vi "WLAN - TV - OPPO - RW - UTIL - TestVectors_11N.vi"(0 "TV_IQComposite_11N":T1={"Standard"=3, "OFDM Advanced Controls"={"OFDM Auto Compute Acquisition Length Enabled"=0, "OFDM Maximum Symbols Used"=0, "OFDM Time Tracking Enabled"=0, "OFDM Channel Tracking Enabled"=0, "OFDM Amplitude Tracking Enabled"=1, "OFDM CFO Estimation Method"=0, "OFDM Phase Tracking Method"=0, "OFDM Header Detection Enabled"=0, "OFDM MAC FCS Check Enabled"=0, "#Avg"=10, "#Iterations"=10}, "Measurement Enabled"=FALSE, "#Packets"=0, "Guard Interval (s)"=0.0, "FEC Coding Type"=0, "80211n PLCP Frame Format"=0, "Generation Parameters"={"Channel Bandwidth(Hz)"=20000000.0, "MCS Index"=0, "OFDM Payload Length (bytes)"=4024, "Idle Interval(S)"=0.0}, "Power Level(dBm)"=0.0, "Center Frequency(Hz)"=0.0} {"Center Frequency(Hz)" format="%#_6p"; "Generation Parameters"."Channel Bandwidth(Hz)" items=["5M"=5000000.0, "10M"=10000000.0, "20M"=20000000.0, "40M"=40000000.0, "80M"=80000000.0, "160M"=160000000.0]; "80211n PLCP Frame Format" items=["Mixed Format", "Greenfield Format"]; "FEC Coding Type" items=["BCC", "LDPC"]; "OFDM Advanced Controls"."OFDM Phase Tracking Method" items=["Standard", "Instantaneous", "None", "Standard with Cubic Spline Fit"]; "OFDM Advanced Controls"."OFDM CFO Estimation Method" items=["Preamble Only", "Preamble and Data"]; "OFDM Advanced Controls"."OFDM Channel Tracking Enabled" items=["False", "True"]; "OFDM Advanced Controls"."OFDM Amplitude Tracking Enabled" items=["False", "True"]; "OFDM Advanced Controls"."OFDM Time Tracking Enabled" items=["True"=1, "False"=0]; "OFDM Advanced Controls"."OFDM Auto Compute Acquisition Length Enabled" items=["False", "True"]; "OFDM Advanced Controls"."OFDM MAC FCS Check Enabled" items=["False", "True"]; "OFDM Advanced Controls"."OFDM Header Detection Enabled" items=["False", "True"]; "Standard" items=["80211A/G/J/P OFDM", "80211B/G DSSS", "80211G DSSSOFDM", "80211N MIMOOFDM", "80211AC MIMOOFDM"]}, 7 "TV Paramaters":T3) -> (6 "TV":string[][](array[string]), 8 "Measure Config":string[][](array[string]))   [LabVIEW 2012]
uses:
  Includes/WLAN - TV - RW - INC - TV_Parameters.ctl
  Includes/WLAN - TV - OPPO - RW - INC - TV_IQComposite_11N.ctl
  Includes/WLAN - TV - RW - INC - TV_OFDM Demod.ctl
  Includes/WLAN - TV - RW - INC - Tx_Meas_Settings_OFDM_String.ctl
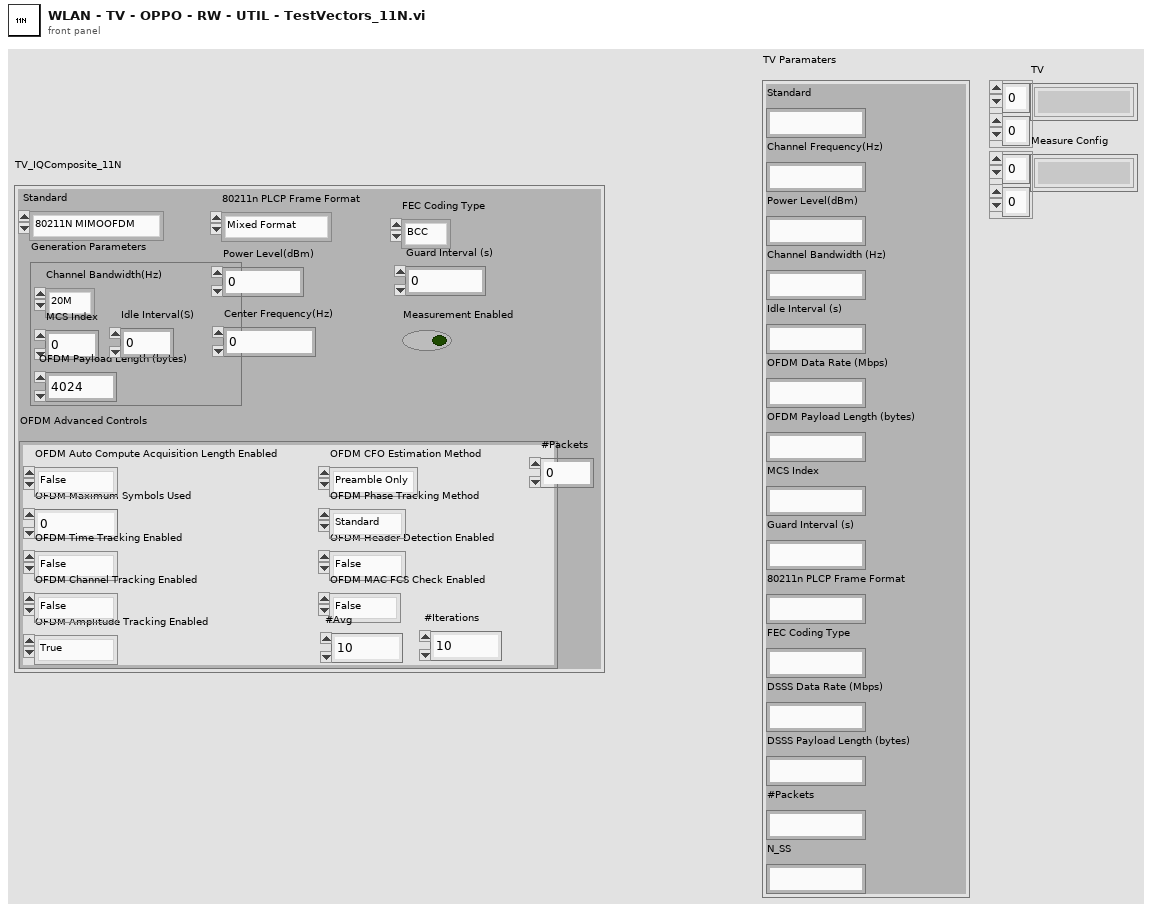
[diagram p1: front panel]
types:
  T1 = typedef "WLAN - TV - OPPO - RW - INC - TV_IQComposite_11N.ctl" = cluster{"Standard":i32, "OFDM Advanced Controls":T2, "Measurement Enabled":bool, "#Packets":i32, "Guard Interval (s)":dbl, "FEC Coding Type":i32, "80211n PLCP Frame Format":i32, "Generation Parameters":cluster{"Channel Bandwidth(Hz)":dbl, "MCS Index":i32, "OFDM Payload Length (bytes)":i32, "Idle Interval(S)":dbl}, "Power Level(dBm)":dbl, "Center Frequency(Hz)":dbl}
  T2 = typedef "WLAN - TV - RW - INC - TV_OFDM Demod.ctl" = cluster{"OFDM Auto Compute Acquisition Length Enabled":i32, "OFDM Maximum Symbols Used":i32, "OFDM Time Tracking Enabled":i32, "OFDM Channel Tracking Enabled":i32, "OFDM Amplitude Tracking Enabled":i32, "OFDM CFO Estimation Method":i32, "OFDM Phase Tracking Method":i32, "OFDM Header Detection Enabled":i32, "OFDM MAC FCS Check Enabled":i32, "#Avg":i32, "#Iterations":i32}
  T3 = typedef "WLAN - TV - RW - INC - TV_Parameters.ctl" = cluster{"Standard ":string, "Channel Frequency(Hz)":string, "Power Level(dBm)":string, "Channel Bandwidth (Hz)":string, "Idle Interval (s)":string, "OFDM Data Rate (Mbps)":string, "OFDM Payload Length (bytes)":string, "MCS Index":string, "Guard Interval (s)":string, "80211n PLCP Frame Format":string, "FEC Coding Type":string, "DSSS Data Rate (Mbps)":string, "DSSS Payload Length (bytes)":string, "#Packets":string, "N_SS":string}
  T4 = typedef "WLAN - TV - RW - INC - Tx_Meas_Settings_OFDM_String.ctl" = cluster{"OFDM Auto Compute Acquisition Length Enabled":string, "OFDM Maximum Symbols Used":string, "OFDM Time Tracking Enabled":string, "OFDM Channel Tracking Enabled":string, "OFDM Amplitude Tracking Enabled":string, "OFDM CFO Estimation Method":string, "OFDM Phase Tracking Method":string, "OFDM Header Detection Enabled":string, "OFDM MAC FCS Check Enabled":string, "#Avg":string, "#Iterations":string}
  T5 = cluster{"Channel Bandwidth(Hz)":dbl, "MCS Index":i32, "OFDM Payload Length (bytes)":i32, "Idle Interval(S)":dbl}
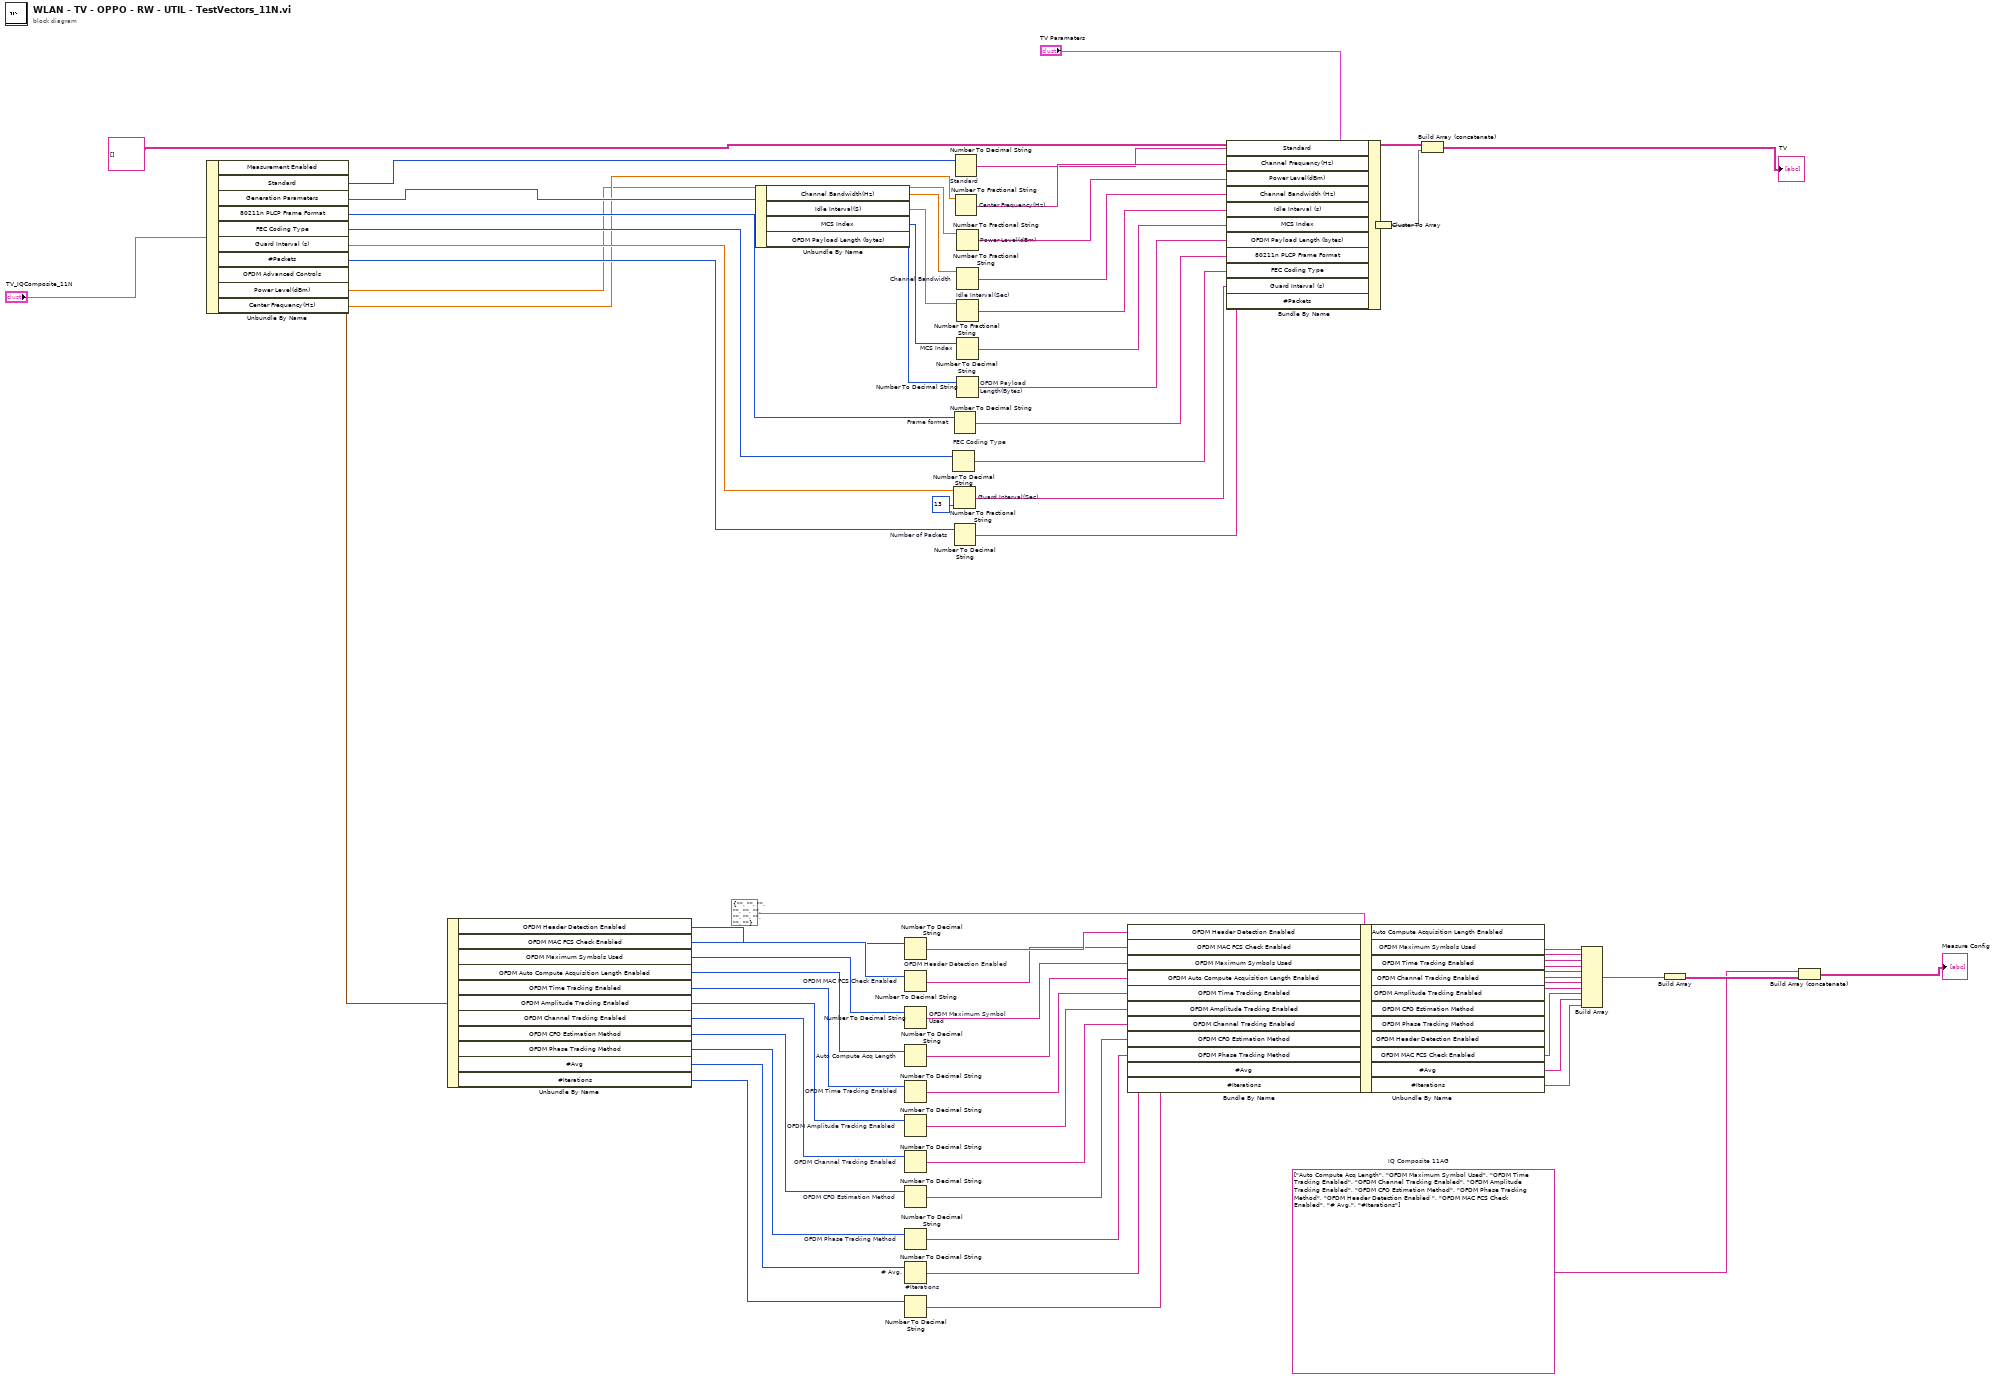
[diagram p0: block diagram]
diagram:
  w24 = string[] ["Auto Compute Acq Length", "OFDM Maximum Symbol Used", "OFDM Time Tracking Enabled", "OFDM Channel Tracking Enabled", "OFDM Amplitude Tracking Enabled", "OFDM CFO Estimation Method", "OFDM Phase Tracking Method", "OFDM Header Detection Enabled ", "OFDM MAC FCS Check Enabled", "# Avg.", "#Iterations"]  # IQ Composite 11AG
  n1 = Unbundle By Name("TV_IQComposite_11N") -> ("Standard"=w68:i32, "Generation Parameters"=w64:T5, "80211n PLCP Frame Format"=w65:i32, "FEC Coding Type"=w70:i32, "Guard Interval (s)"=w69:dbl, "#Packets"=w63:i32, "OFDM Advanced Controls"=w25:T2, "Power Level(dBm)"=w19:dbl, "Center Frequency(Hz)"=w20:dbl)  [unwired: 1 out]
  n2 = Unbundle By Name(w25) -> ("OFDM Header Detection Enabled"=w52:i32, "OFDM MAC FCS Check Enabled"=w53:i32, "OFDM Maximum Symbols Used"=w54:i32, "OFDM Auto Compute Acquisition Length Enabled"=w55:i32, "OFDM Time Tracking Enabled"=w56:i32, "OFDM Amplitude Tracking Enabled"=w57:i32, "OFDM Channel Tracking Enabled"=w58:i32, "OFDM CFO Estimation Method"=w59:i32, "OFDM Phase Tracking Method"=w60:i32, "#Avg"=w61:i32, "#Iterations"=w62:i32)
  n3 = Unbundle By Name(w64) -> ("Channel Bandwidth(Hz)"=w5:dbl, "Idle Interval(S)"=w6:dbl, "MCS Index"=w7:i32, "OFDM Payload Length (bytes)"=w8:i32)
  n4 = Number To Decimal String "OFDM Header Detection Enabled"(number=w52) -> (decimal integer string=w50:string)  [unwired: 1 in]
  n5 = Number To Decimal String "OFDM MAC FCS Check Enabled"(number=w53) -> (decimal integer string=w49:string)  [unwired: 1 in]
  n6 = Number To Decimal String "OFDM Maximum Symbol Used"(number=w54) -> (decimal integer string=w48:string)  [unwired: 1 in]
  n7 = Number To Decimal String "Auto Compute Acq Length"(number=w55) -> (decimal integer string=w47:string)  [unwired: 1 in]
  n8 = Number To Decimal String "OFDM Time Tracking Enabled"(number=w56) -> (decimal integer string=w46:string)  [unwired: 1 in]
  n9 = Number To Decimal String "OFDM Amplitude Tracking Enabled"(number=w57) -> (decimal integer string=w45:string)  [unwired: 1 in]
  n10 = Number To Decimal String "OFDM Channel Tracking Enabled"(number=w58) -> (decimal integer string=w40:string)  [unwired: 1 in]
  n11 = Number To Decimal String "OFDM CFO Estimation Method"(number=w59) -> (decimal integer string=w41:string)  [unwired: 1 in]
  n12 = Number To Decimal String "OFDM Phase Tracking Method"(number=w60) -> (decimal integer string=w42:string)  [unwired: 1 in]
  n13 = Number To Decimal String "# Avg."(number=w61) -> (decimal integer string=w43:string)  [unwired: 1 in]
  n14 = Number To Decimal String "#Iterations"(number=w62) -> (decimal integer string=w44:string)  [unwired: 1 in]
  n15 = Number To Decimal String "FEC Coding Type"(number=w70) -> (decimal integer string=w9:string)  [unwired: 1 in]
  n16 = Number To Fractional String "Guard Interval(Sec)"(number=w69, precision (6)=i16 13) -> (F-format string=w10:string)  [unwired: 2 in]
  n17 = Number To Decimal String "Frame format"(number=w65) -> (decimal integer string=w11:string)  [unwired: 1 in]
  n18 = Number To Decimal String "Number of Packets"(number=w63) -> (decimal integer string=w4:string)  [unwired: 1 in]
  n19 = Number To Decimal String "Standard"(number=w68) -> (decimal integer string=w12:string)  [unwired: 1 in]
  n20 = Number To Fractional String "Center Frequency(Hz)"(number=w20) -> (F-format string=w13:string)  [unwired: 3 in]
  n21 = Number To Fractional String "Power Level(dBm)"(number=w19) -> (F-format string=w14:string)  [unwired: 3 in]
  n22 = Number To Fractional String "Channel Bandwidth"(number=w5) -> (F-format string=w15:string)  [unwired: 3 in]
  n23 = Number To Fractional String "Idle Interval(Sec)"(number=w6) -> (F-format string=w16:string)  [unwired: 3 in]
  n24 = Number To Decimal String "MCS Index"(number=w7) -> (decimal integer string=w17:string)  [unwired: 1 in]
  n25 = Number To Decimal String "OFDM Payload Length(Bytes)"(number=w8) -> (decimal integer string=w18:string)  [unwired: 1 in]
  n26 = Bundle By Name(cluster=T4 {"OFDM Auto Compute Acquisition Length Enabled"="", "OFDM Maximum Symbols Used"="", "OFDM Time Tracking Enabled"="", "OFDM Channel Tracking Enabled"="", "OFDM Amplitude Tracking Enabled"="", "OFDM CFO Estimation Method"="", "OFDM Phase Tracking Method"="", "OFDM Header Detection Enabled"="", "OFDM MAC FCS Check Enabled"="", "#Avg"="", "#Iterations"=""} ("OFDM Measurement Settings"), "OFDM Header Detection Enabled"=w50, "OFDM MAC FCS Check Enabled"=w49, "OFDM Maximum Symbols Used"=w48, "OFDM Auto Compute Acquisition Length Enabled"=w47, "OFDM Time Tracking Enabled"=w46, "OFDM Amplitude Tracking Enabled"=w45, "OFDM Channel Tracking Enabled"=w40, "OFDM CFO Estimation Method"=w41, "OFDM Phase Tracking Method"=w42, "#Avg"=w43, "#Iterations"=w44) -> (w39:T4)
  n27 = Bundle By Name(cluster="TV Paramaters", "Standard"=w12, "Channel Frequency(Hz)"=w13, "Power Level(dBm)"=w14, "Channel Bandwidth (Hz)"=w15, "Idle Interval (s)"=w16, "MCS Index"=w17, "OFDM Payload Length (bytes)"=w18, "80211n PLCP Frame Format"=w11, "FEC Coding Type"=w9, "Guard Interval (s)"=w10, "#Packets"=w4) -> (w2:T3)
  n28 = Unbundle By Name(w39) -> ("OFDM Auto Compute Acquisition Length Enabled"=w38:string, "OFDM Maximum Symbols Used"=w37:string, "OFDM Time Tracking Enabled"=w36:string, "OFDM Channel Tracking Enabled"=w35:string, "OFDM Amplitude Tracking Enabled"=w34:string, "OFDM CFO Estimation Method"=w33:string, "OFDM Phase Tracking Method"=w32:string, "OFDM Header Detection Enabled"=w31:string, "OFDM MAC FCS Check Enabled"=w30:string, "#Avg"=w29:string, "#Iterations"=w28:string)
  n29 = Cluster To Array(cluster=w2) -> (array=w1:string[])
  n30 = Build Array (concatenate)(string[][] [] ("appended array"), w1) -> (→"TV":string[][])
  n31 = Build Array(w38, w37, w36, w35, w34, w33, w32, w31, w30, w29, w28) -> (w27:string[])
  n32 = Build Array(w27) -> (w26:string[][])
  n33 = Build Array (concatenate)(w24, w26) -> (→"Measure Config":string[][])
